vi "insert_component.vi"(8 "error in (no error)":errorcluster, 9 "who":string, 10 "Component":T1, 11 "DB Session ID":i32) -> (0 "error out":errorcluster, 2 "Component out":T1, 3 "DB Session ID out":i32)   [LabVIEW 2023, in "Database.lvlib"]
uses:
  Database.lvlib
  DB Component.ctl
  bin/Database.dll
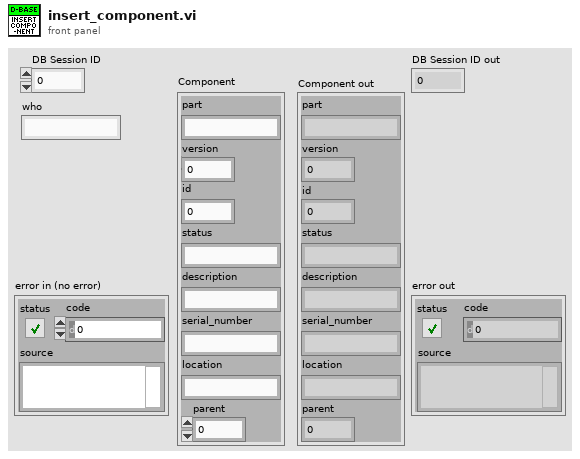
[diagram p1: front panel]
types:
  T1 = typedef "Database.lvlib/DB Component.ctl" = cluster{"part":string, "version":i32, "id":i32, "status":string, "description":string, "serial_number":string, "location":string, "parent":i32}
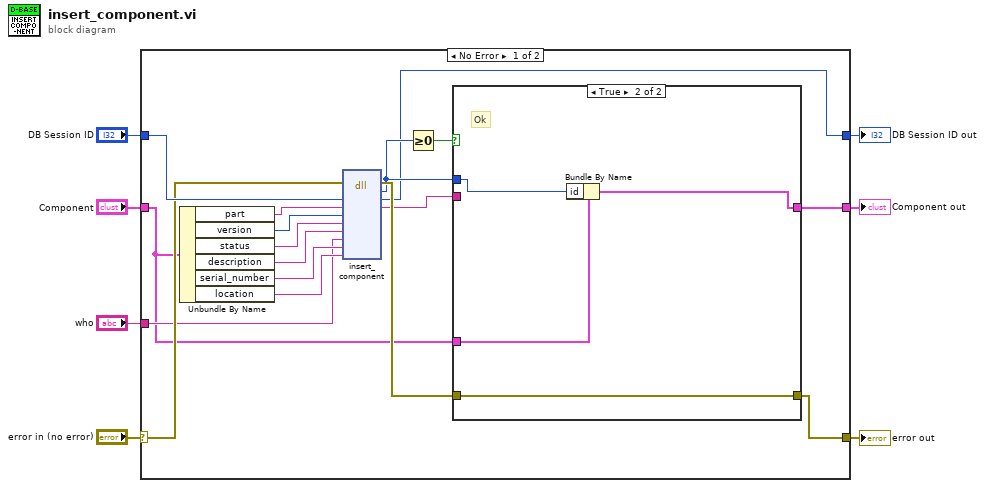
[diagram p0: block diagram]
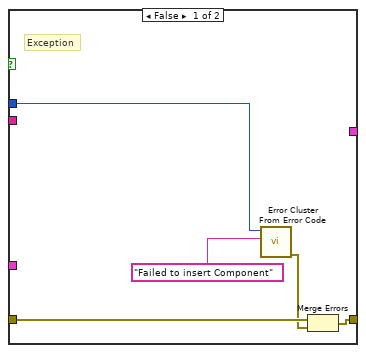
[diagram p2: hidden frame]
diagram:
  n1 = case shown="No Error" "error in (no error)" {
    selector: "error in (no error)" -> [w22 w36]
    tunnel: [w21 w36] -> w5
    tunnel: "DB Session ID" -> [w23 w35]
    tunnel: [w18 w34] -> w1
    tunnel: [w16 w35] -> w4
    tunnel: "Component" -> [w8 w34]
    tunnel: "who" -> [w9 _]
    frame No Error {
      n2 = Unbundle By Name(w8) -> ("part"=w15:string, "version"=w14:i32, "status"=w13:string, "description"=w12:string, "serial_number"=w11:string, "location"=w10:string)
      n3 = dll-call lib="C:/Users/cfangmeier3/Desktop/nebraska-silicon-lab/pixel-gantry-control/Gantry/Shared Components/bin/Database.dll" fn="insert_component"(error in=w22, "conn_id"=w23, "part"=w15, "version"=w14, "status"=w13, "description"=w12, "who"=w9, "serial_number"=w11, "location"=w10) -> (error out=w24:errorcluster, "return type"=w17:i32, "conn_id"=w16:i32, "part"=w19:string)  [unwired: 8 in, 1 out]
      n4 = Greater Or Equal To 0?(x=w17) -> (x >= 0?=w20:bool)
      n5 = case shown="True" w20 {
        tunnel: w24 -> [w29 w33]
        tunnel: [w28 w33] -> w21
        tunnel: w19 -> [_ _]
        tunnel: [_ w30] -> w18
        tunnel: w17 -> [w25 w31]
        tunnel: w8 -> [_ w32]
        frame False {
          # "Exception"
          n6 = call <vilib>:"Error Cluster From Error Code.vi"("error message (\"\")"="Failed to insert Component" ("error message (\"\")"), "error code (0)"=w25) -> ("error out"=w27:errorcluster)  [unwired: 7 in]
          n7 = Merge Errors(w29, w27) -> (w28:errorcluster)
        }
        frame True {
          # "Ok"
          n8 = Bundle By Name(cluster=w32, "id"=w31) -> (w30:T1)
        }
      }
    }
    frame Error {
    }
  }
  "error out" <- w5
  "DB Session ID out" <- w4
  "Component out" <- w1
